vi "Main.vi"() -> ()   [LabVIEW 2021]
uses:
  <vilib>/FPGAPlugInAG/myRIO-1900/niLvFpga_Open_myRIO-1900.vi
  <vilib>/rvi/interface/common/dynamic/niFpgaDynamicAddResources.vi
  <vilib>/Utility/error.llb/Error Cluster From Error Code.vi
  <vilib>/rvi/errors/niLvFpgaAdjustHostInterfaceError.vi
  <vilib>/FPGAPlugInAG/Dynamic/niLvFpga_Close_Dynamic.vi
  <vilib>/rvi/interface/nirviOpenFPGA/nirviOpenFPGA.xnode
  FPGA Bitfiles/fpga-rtandfpga-h_FPGATarget_FPGAMain_XFpyvtSvrYk.lvbitx
  <vilib>/rvi/interface/nirviReadWriteControl/nirviReadWriteControl.xnode
  <vilib>/rvi/interface/nirviCloseFPGA/nirviCloseFPGA.xnode
  NiFpgaLv.dll
  <vilib>/rvi/interface/Simulation/niFpgaSimulationCallBeginRW.vi
panel:
  in  "stop":bool
  out "Button0":bool
  in  "Led0":bool
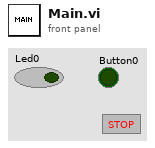
[diagram p1: front panel]
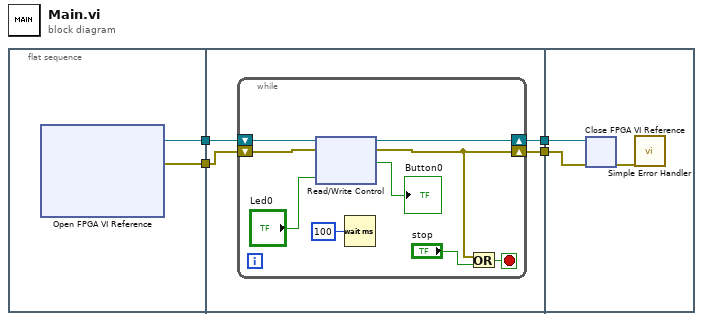
[diagram p0: block diagram]
diagram:
  n1 = flat-sequence {
    tunnel: [w6] -> w4
    tunnel: [w5] -> w2
    tunnel: w4 -> [w10]
    tunnel: [w9] -> w3
    tunnel: w2 -> [w8]
    tunnel: [w7] -> w1
    tunnel: w3 -> [w22]
    tunnel: w1 -> [w21]
    frame #0 {
      n2 = xnode "Open FPGA VI Reference"() -> ("FPGA VI Reference Out"=w6:refnum<k20>, "error out"=w5:errorcluster)  [unwired: 2 in]
    }
    frame #1 {
      n3 = while {
        shift-right: [w18] -> w9
        shift-left: w10 -> [w19]
        shift-right: [w12] -> w7
        shift-left: w8 -> [w17]
        stop <- w13 stop-if-true
        n4 = xnode "Read/Write Control"("FPGA VI Reference In"=w19, "error in"=w17, "Led0"="Led0") -> ("FPGA VI Reference Out"=w18:refnum<k20>, "error out"=w12:errorcluster, "Button0"=→"Button0":bool)
        n5 = Wait (ms)(milliseconds to wait=u32 100) -> ()  [unwired: 1 out]
        n6 = Or(x=w12, y="stop") -> (x .or. y?=w13:bool)
      }
    }
    frame #2 {
      n7 = xnode "Close FPGA VI Reference"("FPGA VI Reference In"=w22, "error in"=w21) -> ("error out"=w20:errorcluster)
      n8 = call <vilib>:"Simple Error Handler.vi"("error in (no error)"=w20) -> ()  [unwired: 4 in, 5 out]
    }
  }
